vi "PPL_Main Page.vi"(8 "error in (no error)":errorcluster, 11 "Node Ptr":T1 format="%.0x") -> (0 "error out":errorcluster)   [LabVIEW 2020]
uses:
  <vilib>/NI VeriStand/Custom Device API/Custom Device API.lvlib
  <vilib>/NI VeriStand/Custom Device API/Custom Device Item Ref.ctl
panel:
  out "Version":string
  in  "SHDocVw.IWebBrowser":refnum<k7>(container)
  in  "Specific Header":cluster{"Section Name":string}={"Section Name"="Custom Device Item Settings"}
  in  "General Header":cluster{"Section Name":string}={"Section Name"="General Custom Device Settings"}
  in  "Description":string
  in  "Name":string
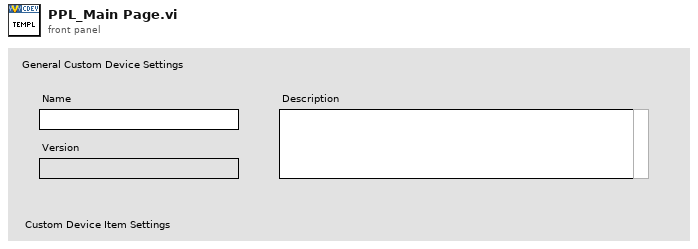
[diagram p1: front panel]
types:
  T1 = typedef "Custom Device API.lvlib/Custom Device Item Ref.ctl" = u64
  T2 = typedef "Custom Device API.lvlib/Custom Device Item Info.ctl" = cluster{"Name":string, "Is Channel":bool, "GUID":string, "Is Waveform":bool}
  T3 = typedef "Custom Device API.lvlib/Custom Device Commands.ctl" = enum16{"Default", "Item renamed", "Shutdown", "Dynamic button pressed"}
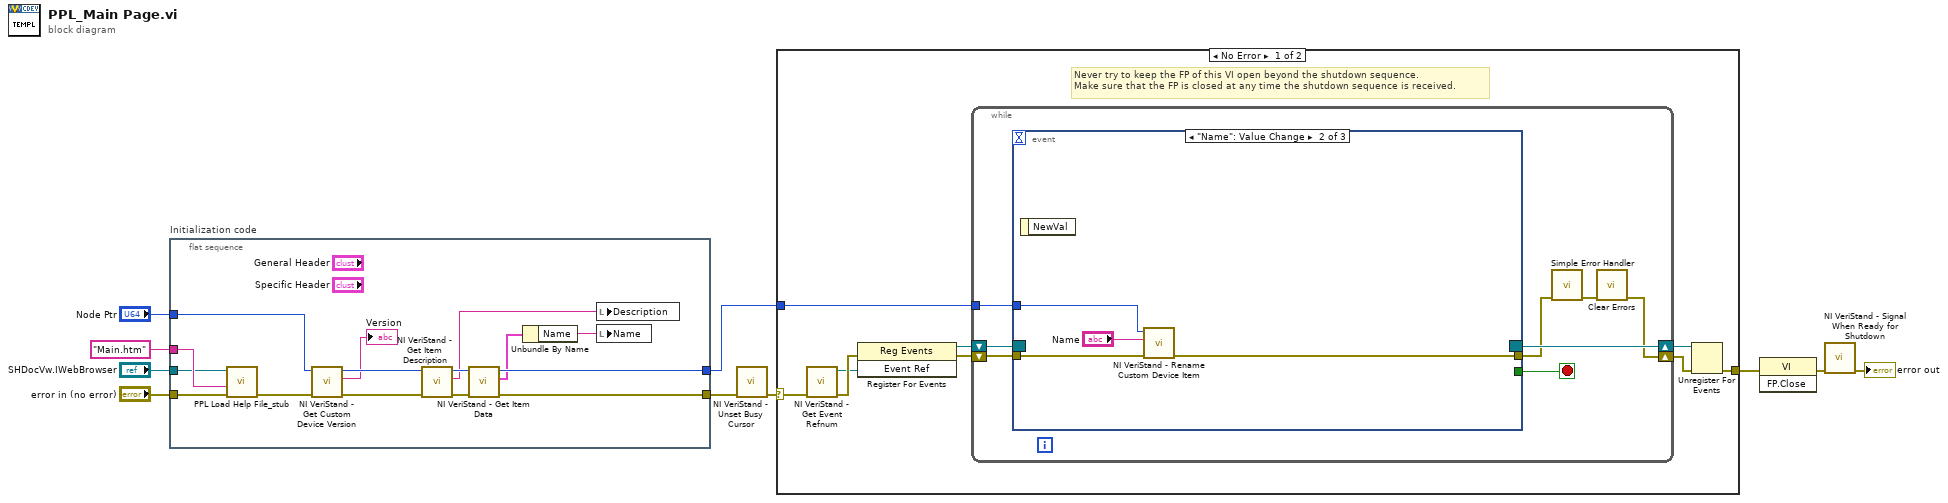
[diagram p0: block diagram]
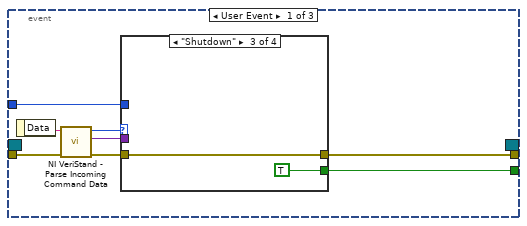
[diagram p2: hidden frame]
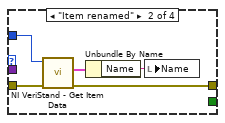
[diagram p4: hidden frame]
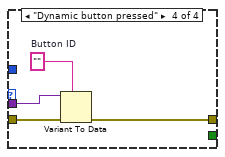
[diagram p5: hidden frame]
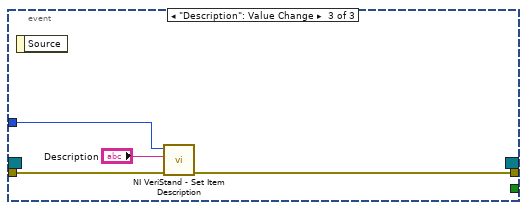
[diagram p6: hidden frame]
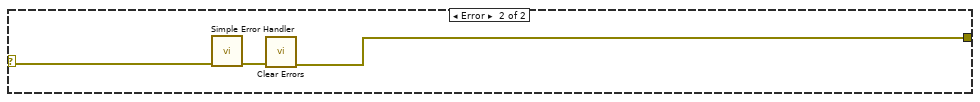
[diagram p7: hidden frame]
diagram:
  n1 = flat-sequence "Initialization code" {
    tunnel: "error in (no error)" -> [w14]
    tunnel: "Node Ptr" -> [w20]
    tunnel: [w21] -> w6
    tunnel: [w25] -> w3
    tunnel: "SHDocVw.IWebBrowser" -> [w11]
    tunnel: "Main.htm" ("HTML File") -> [w12]
    frame #0 {
      n2 = call "PPL Load Help File_stub.vi"("error in (no error)"=w14, "HTML File to Load"=w12, "Browser"=w11) -> ("error out"=w13:errorcluster)  [unwired: 8 in]
      n3 = call <vilib>:"NI VeriStand - Get Custom Device Version.vi"("error in (no error)"=w13, "Device Ref in"=w20) -> ("error out"=w19:errorcluster, "Value"=→"Version":string, "Device Ref out"=w18:T1)  [unwired: 7 in]
      n4 = call <vilib>:"NI VeriStand - Get Item Description.vi"("error in (no error)"=w19, "Item Ref in"=w18) -> ("error out"=w23:errorcluster, "Description"=w15:string, "Item Ref out"=w24:T1)  [unwired: 7 out]
      n5 = call <vilib>:"NI VeriStand - Get Item Data.vi"("error in (no error)"=w23, "Item Ref in"=w24) -> ("error out"=w21:errorcluster, "Item Info"=w22:T2, "Item Ref out"=w25:T1)  [unwired: 7 out]
      n6 = Unbundle By Name(w22) -> ("Name"=w16:string)
      n7 = local write "Description"(w15) -> ()
      n8 = local write "Name"(w16) -> ()
    }
  }
  n9 = call <vilib>:"NI VeriStand - Unset Busy Cursor.vi"("error in (no error)"=w6) -> ("error out"=w5:errorcluster)  [unwired: 10 out]
  n10 = case shown="No Error" w5 {
    selector: w5 -> [w26 w73]
    tunnel: [w31 w71] -> w10
    tunnel: w3 -> [w27 _]
    frame No Error {
      # "Never try to keep the FP of this VI open beyond the shutdown sequence.\nMake sure that the FP is closed at any time the shutdown sequence is received."
      n11 = call <vilib>:"NI VeriStand - Get Event Refnum.vi"("error in (no error)"=w26) -> ("error out"=w34:errorcluster, "Event Ref"=w30:refnum<user-event>)  [unwired: 9 out]
      n12 = register-events(error in=w34, w30) -> (reference out=w28:refnum<event-registration>, error out=w29:errorcluster)  [unwired: 1 in]
      n13 = while {
        tunnel: w27 -> [w38]
        shift-right: [w35] -> w32
        shift-left: w29 -> [w41]
        shift-right: [w42] -> w33
        shift-left: w28 -> [w40]
        stop <- w39 stop-if-true
        n14 = event shown="[1] \"Name\": Value Change" {
          selector: w40 -> [_ _ _]
          dyn-events: [_ _ _] -> w42
          timeout: _ -> [_ _ _]
          tunnel: w41 -> [w50 w66 w69]
          tunnel: [w46 _ _] -> w39
          tunnel: [w45 w65 w68] -> w37
          tunnel: w38 -> [w44 w64 w70]
          event User Event {
            n15 = event-data() -> ("Data"=w49:string)  [unwired: 1 out]
            n16 = call <vilib>:"NI VeriStand - Parse Incoming Command Data.vi"("error in (no error)"=w50, "Incoming data"=w49) -> ("error out"=w48:errorcluster, "Outgoing data"=w43:variant, "Action"=w47:T3)  [unwired: 7 out]
            n17 = case shown="\"Shutdown\"" w47 {
              tunnel: w48 -> [w51 w56 w57 w62]
              tunnel: [_ _ TRUE _] -> w46
              tunnel: [w51 w53 w57 w59] -> w45
              tunnel: w44 -> [_ w55 _ _]
              tunnel: w43 -> [_ _ _ w61]
              frame "Default", Default {
              }
              frame "Item renamed" {
                n18 = call <vilib>:"NI VeriStand - Get Item Data.vi"("error in (no error)"=w56, "Item Ref in"=w55) -> ("error out"=w53:errorcluster, "Item Info"=w54:T2)  [unwired: 8 out]
                n19 = Unbundle By Name(w54) -> ("Name"=w52:string)
                n20 = local write "Name"(w52) -> ()
              }
              frame "Shutdown" {
              }
              frame "Dynamic button pressed" {
                w60 = ""  # Button ID
                n21 = Variant To Data(error in=w62, type=w60, Variant=w61) -> (error out=w59:errorcluster)  [unwired: 1 out]
              }
            }
          }
          event "Name": Value Change {
            n22 = event-data() -> ()  [unwired: 2 out]
            n23 = call <vilib>:"NI VeriStand - Rename Custom Device Item.vi"("error in (no error)"=w66, "New Name"="Name", "Item Ref in"=w64) -> ("error out"=w65:errorcluster)  [unwired: 1 in, 7 out]
          }
          event "Description": Value Change {
            n24 = event-data() -> ()  [unwired: 2 out]
            n25 = call <vilib>:"NI VeriStand - Set Item Description.vi"("error in (no error)"=w69, "Description"="Description", "Item Ref in"=w70) -> ("error out"=w68:errorcluster)  [unwired: 8 out]
          }
        }
        n26 = call <vilib>:"Simple Error Handler.vi"("error in (no error)"=w37) -> ("error out"=w36:errorcluster)  [unwired: 1 in, 7 out]
        n27 = call <vilib>:"Clear Errors.vi"("error in (no error)"=w36) -> ("error out"=w35:errorcluster)  [unwired: 1 in, 5 out]
      }
      n28 = Unregister For Events(event registration refnum=w33, error in=w32) -> (error out=w31:errorcluster)
    }
    frame Error {
      n29 = call <vilib>:"Simple Error Handler.vi"("error in (no error)"=w73) -> ("error out"=w72:errorcluster)  [unwired: 1 in, 7 out]
      n30 = call <vilib>:"Clear Errors.vi"("error in (no error)"=w72) -> ("error out"=w71:errorcluster)  [unwired: 1 in, 5 out]
    }
  }
  n31 = invoke class="VI" method="FP.Close"(error in=w10) -> (error out=w9:errorcluster)  [unwired: 2 in, 2 out]
  n32 = call <vilib>:"NI VeriStand - Signal When Ready for Shutdown.vi"("error in (no error)"=w9) -> ("error out"=→"error out":errorcluster)  [unwired: 10 out]
